vi "SFOAE-Create Compensated Sweep.vi"(0 "Sweep":T1, 2 "Overlap (kHz)":dbl, 5 "Level (dB SPL)":dbl, 7 "Cal File":path, 9 "Fs (Hz)":dbl, 11 "error in (no error)":errorcluster) -> (4 "sweep":dbl[](array[numeric]), 6 "RampPts":i32, 8 "offset":i32, 15 "error out":errorcluster)   [LabVIEW 2020]
uses:
  Typedefs/SFOAE-Sweep Params.ctl
  epl-vi-lib/Utility VIs/Math VIs/LinSpace (x0-dx-npts).vi
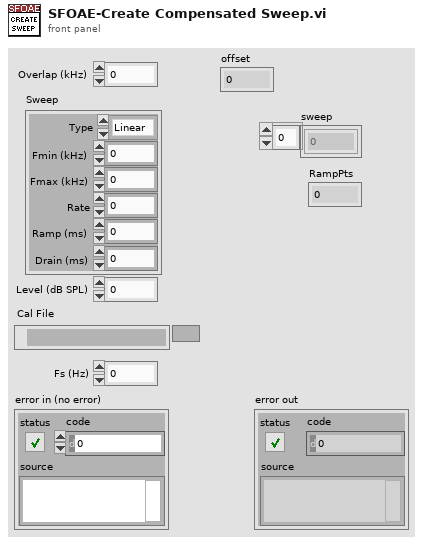
[diagram p1: front panel]
types:
  T1 = typedef "SFOAE-Sweep Params.ctl" = cluster{"Type":enum16{"Linear", "Log"}, "Fmin (kHz)":dbl, "Fmax (kHz)":dbl, "Rate":dbl, "Ramp (ms)":dbl, "Drain (ms)":dbl}
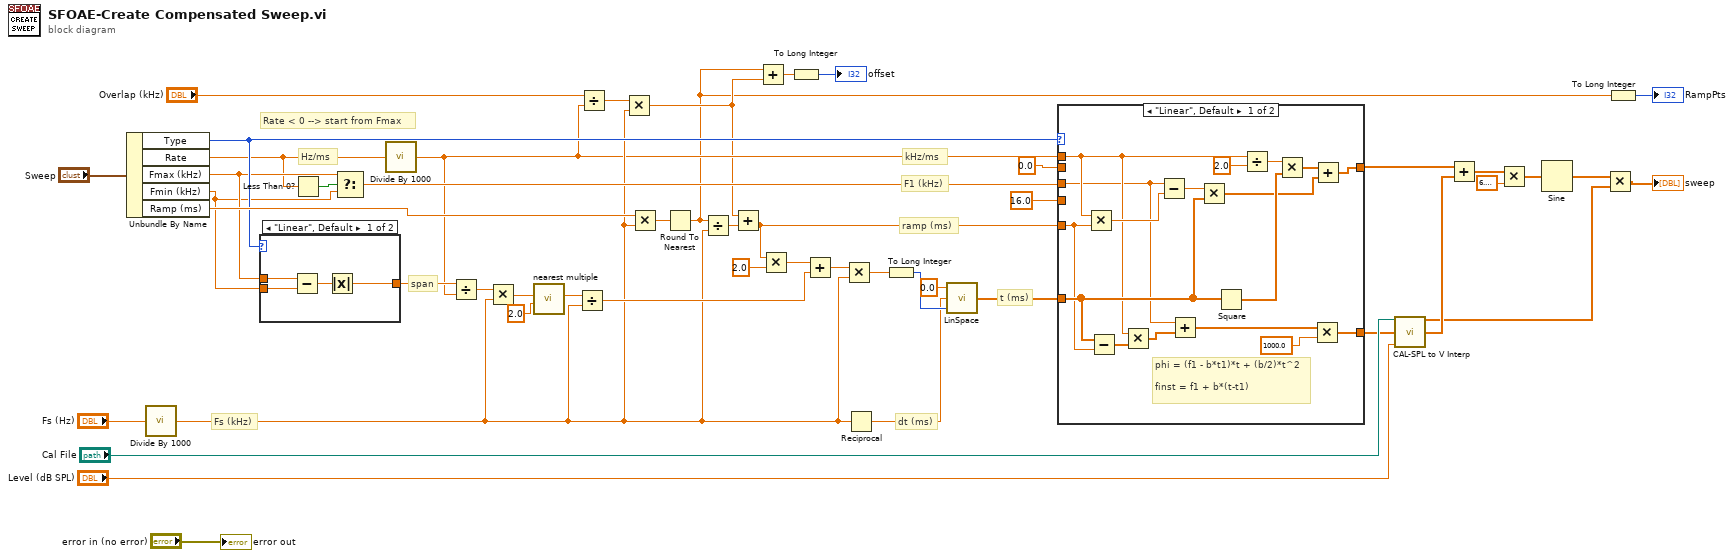
[diagram p0: block diagram]
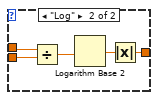
[diagram p3: hidden frame]
diagram:
  # "Hz/ms"
  # "Rate < 0 --> start from Fmax"
  # "F1 (kHz)"
  # "kHz/ms"
  # "ramp (ms)"
  # "t (ms)"
  # "dt (ms)"
  # "Fs (kHz)"
  # "span"
  n1 = Unbundle By Name("Sweep") -> ("Type"=w33:enum16{"Linear", "Log"}, "Rate"=w26:dbl, "Fmax (kHz)"=w31:dbl, "Fmin (kHz)"=w30:dbl, "Ramp (ms)"=w44:dbl)
  n2 = call "Divide By 1000.vi"("X"="Fs (Hz)") -> ("X/1000"=w9:dbl)
  n3 = case shown="\"Linear\", Default" w33 {
    tunnel: w31 -> [w53 w57]
    tunnel: w30 -> [w52 w58]
    tunnel: [w50 w55] -> w49
    frame "Linear", Default {
      n4 = Subtract(x=w53, y=w52) -> (x-y=w51:dbl)
      n5 = Absolute Value(x=w51) -> (abs(x)=w50:dbl)
    }
    frame "Log" {
      n6 = Divide(x=w57, y=w58) -> (x/y=w56:dbl)
      n7 = Logarithm Base 2(1:w56) -> (0:w54:dbl)
      n8 = Absolute Value(x=w54) -> (abs(x)=w55:dbl)
    }
  }
  n9 = Less Than 0?(x=w26) -> (x < 0?=w32:bool)
  n10 = Select(t=w31, s=w32, f=w30) -> (s? t:f=w29:dbl)
  n11 = call "Divide By 1000.vi"("X"=w26) -> ("X/1000"=w5:dbl)
  n12 = Divide(x=w49, y=w5) -> (x/y=w48:dbl)
  n13 = Multiply(x=w48, y=w9) -> (x*y=w47:dbl)
  n14 = call "nearest multiple.vi"("y"=2.0, "x"=w47) -> ("round(x/y)*y"=w45:dbl)  [unwired: 7 in, 2 out]
  n15 = Divide(x=w45, y=w9) -> (x/y=w40:dbl)
  n16 = Divide(x="Overlap (kHz)", y=w5) -> (x/y=w7:dbl)
  n17 = Multiply(x=w7, y=w9) -> (x*y=w4:dbl)
  n18 = Multiply(x=w44, y=w9) -> (x*y=w43:dbl)
  n19 = Round To Nearest(number=w43) -> (nearest integer value=w3:dbl)
  n20 = Divide(x=w3, y=w9) -> (x/y=w24:dbl)
  n21 = Add(x=w4, y=w24) -> (x+y=w8:dbl)
  n22 = Add(x=w3, y=w4) -> (x+y=w2:dbl)
  n23 = Multiply(x=w8, y=2.0) -> (x*y=w41:dbl)
  n24 = To Long Integer(number=w2) -> (32bit integer=→"offset":i32)
  n25 = Add(x=w41, y=w40) -> (x+y=w39:dbl)
  n26 = Multiply(x=w39, y=w9) -> (x*y=w37:dbl)
  n27 = Reciprocal(x=w9) -> (1/x=w35:dbl)
  n28 = To Long Integer(number=w37) -> (32bit integer=w36:i32)
  n29 = call-poly "LinSpace.vi"("npts"=w36, "dx"=w35, "x0"=0.0) -> ("Array"=w14:dbl[])  [unwired: 1 in, 1 out]
  n30 = case shown="\"Linear\", Default" w33 {
    tunnel: w14 -> [w72 _]
    tunnel: w8 -> [w65 _]
    tunnel: w5 -> [w60 _]
    tunnel: w29 -> [w59 _]
    tunnel: [w62 _] -> w11
    tunnel: [w63 _] -> w13
    tunnel: 0.0 -> [_ _]
    tunnel: 16.0 -> [_ _]
    frame "Linear", Default {
      # "phi = (f1 - b*t1)*t + (b/2)*t^2\n\nfinst = f1 + b*(t-t1)"
      n31 = Multiply(x=w60, y=w65) -> (x*y=w75:dbl)
      n32 = Subtract(x=w72, y=w65) -> (x-y=w66:dbl[])
      n33 = Multiply(x=w60, y=w66) -> (x*y=w67:dbl[])
      n34 = Subtract(x=w59, y=w75) -> (x-y=w74:dbl)
      n35 = Add(x=w59, y=w67) -> (x+y=w64:dbl[])
      n36 = Multiply(x=w74, y=w72) -> (x*y=w68:dbl[])
      n37 = Square(x=w72) -> (x^2=w70:dbl[])
      n38 = Divide(x=w60, y=2.0) -> (x/y=w71:dbl)
      n39 = Multiply(x=w71, y=w70) -> (x*y=w69:dbl[])
      n40 = Multiply(x=w64, y=1000.0) -> (x*y=w62:dbl[])
      n41 = Add(x=w69, y=w68) -> (x+y=w63:dbl[])
    }
    frame "Log" {
    }
  }
  n42 = call "CAL-SPL to V Interp.vi"("user path"="Cal File", "Fi (Hz)"=w11, "dB SPL"="Level (dB SPL)") -> ("Amplitude (V)"=w19:dbl[], "Phase (cycles)"=w20:dbl[])  [unwired: 11 in]
  n43 = Add(x=w13, y=w20) -> (x+y=w21:dbl[])
  n44 = Multiply(x=w21, y=6.283185307179586) -> (x*y=w27:dbl[])
  n45 = Sine(x=w27) -> (sin(x)=w25:dbl[])
  n46 = Multiply(x=w25, y=w19) -> (x*y=→"sweep":dbl[])
  n47 = To Long Integer(number=w3) -> (32bit integer=→"RampPts":i32)
  "error out" <- "error in (no error)"
